vi "Leitura_transdutores_pressão_atualizado.vi"() -> ()   [LabVIEW 2019]
uses:
  <vilib>/Analysis/NI_AALBase.lvlib
panel:
  out "Intermed":dbl format="%0.4f"
  in  "stop":bool
  out "Descarga A0":dbl format="%0.4f"
  out "Sucção A1":dbl format="%0.4f"
  out "XY Graph":cluster{dbl[], dbl[]}[](graph)
  out "Descarga/Sucção":dbl
  in  "Zerar":bool
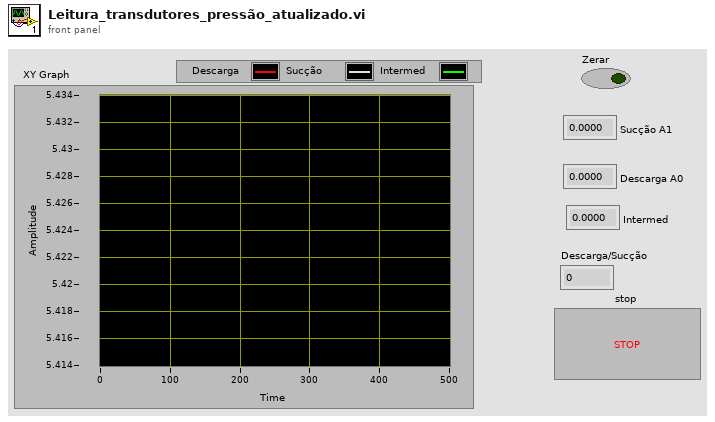
[diagram p1: front panel]
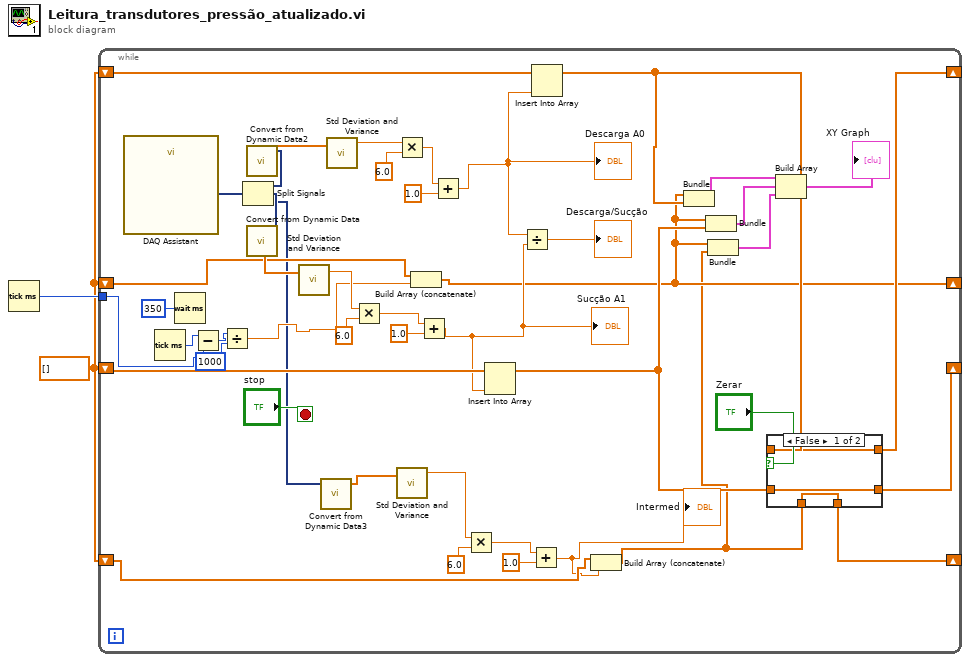
[diagram p0: block diagram]
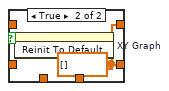
[diagram p2: hidden frame]
diagram:
  w1 = dbl[] []
  n1 = Tick Count (ms)() -> (millisecond timer value=w2:u32)
  n2 = while {
    shift-right: [w33] -> _
    shift-left: w1 -> [w42]
    shift-right: [w34] -> _
    shift-left: w1 -> [w41]
    shift-right: [w8] -> _
    shift-left: w1 -> [w24]
    tunnel: w2 -> [w15]
    shift-right: [w3] -> _
    shift-left: w1 -> [w6]
    stop <- "stop" stop-if-true
    n3 = call "DAQ Assistant"() -> ("data"=w47:dynamicdata)  [unwired: 17 in, 2 out]
    n4 = Tick Count (ms)() -> (millisecond timer value=w17:u32)
    n5 = Wait (ms)(milliseconds to wait=u32 350) -> ()  [unwired: 1 out]
    n6 = Subtract(x=w17, y=w15) -> (x-y=w16:u32)
    n7 = Divide(x=w16, y=u32 1000) -> (x/y=w18:dbl)
    n8 = Split Signals(w47) -> (w45:dynamicdata, w46:dynamicdata, w14:dynamicdata)  [unwired: 3 in]
    n9 = call "Convert from Dynamic Data2"("Dynamic Data Type"=w45) -> ("Array"=w44:dbl[])  [unwired: 3 in]
    n10 = call "Convert from Dynamic Data"("Dynamic Data Type"=w46) -> ("Array"=w43:dbl[])  [unwired: 3 in]
    n11 = call <vilib>:"Std Deviation and Variance.vi"("X"=w43) -> ("mean"=w37:dbl)  [unwired: 1 in, 2 out]
    n12 = call "Convert from Dynamic Data3"("Dynamic Data Type"=w14) -> ("Array"=w13:dbl[])  [unwired: 3 in]
    n13 = call <vilib>:"Std Deviation and Variance.vi"("X"=w44) -> ("mean"=w39:dbl)  [unwired: 1 in, 2 out]
    n14 = Multiply(x=w37, y=6.0) -> (x*y=w30:dbl)
    n15 = Multiply(x=w39, y=6.0) -> (x*y=w29:dbl)
    n16 = call <vilib>:"Std Deviation and Variance.vi"("X"=w13) -> ("mean"=w9:dbl)  [unwired: 1 in, 2 out]
    n17 = Build Array (concatenate)(w24, w18) -> (w8:dbl[])
    n18 = Add(x=w30, y=1.0) -> (x+y=w25:dbl)
    "Sucção A1" <- w25
    n19 = Add(x=w29, y=1.0) -> (x+y=w26:dbl)
    "Descarga A0" <- w26
    n20 = Multiply(x=w9, y=6.0) -> (x*y=w12:dbl)
    n21 = Insert Into Array(array=w41, new element=w25) -> (w23:dbl[])  [unwired: 1 in]
    n22 = Divide(x=w26, y=w25) -> (x/y=→"Descarga/Sucção":dbl)
    n23 = Add(x=w12, y=1.0) -> (x+y=w5:dbl)
    "Intermed" <- w5
    n24 = Insert Into Array(array=w42, new element=w26) -> (w22:dbl[])  [unwired: 1 in]
    n25 = Build Array (concatenate)(w6, w5) -> (w4:dbl[])
    n26 = Bundle(w8, w22) -> (w21:cluster{dbl[], dbl[]})  [unwired: 1 in]
    n27 = Bundle(w8, w23) -> (w20:cluster{dbl[], dbl[]})  [unwired: 1 in]
    n28 = Bundle(w8, w4) -> (w7:cluster{dbl[], dbl[]})  [unwired: 1 in]
    n29 = case shown="False" "Zerar" {
      tunnel: w23 -> [w51 _]
      tunnel: [w51 w52] -> w34
      tunnel: w22 -> [w50 _]
      tunnel: [w50 w52] -> w33
      tunnel: w4 -> [w49 _]
      tunnel: [w49 w52] -> w3
      frame False {
      }
      frame True {
        w52 = dbl[] []
        n30 = invoke on="XY Graph" class="XYGraph (strict)" method="Reinit To Default"() -> ()  [unwired: 3 in, 3 out]
      }
    }
    n31 = Build Array(w21, w20, w7) -> (→"XY Graph":cluster{dbl[], dbl[]}[])
  }
